vi "pannel-test.vi"() -> ()   [LabVIEW 2019]
uses:
  <vilib>/JDP Science/JSONtext/support/Format JSON Object.vi
  <vilib>/addons/Tools/Unicode/UTF8 Tools.lvlib
  <vilib>/JDP Science/JSONtext/JSONtext.lvlib
panel:
  out "<JSON>":string caption="<JSON>Array"
  out "数组 3":string[][](array[string])
  in  "pannel-list":T1(array[cluster])=[{"node"=[{"ID"="1", "Attribute"="dev", "Action"="", "name"="台灯"}, {"ID"="2", "Attribute"="dev", "Action"="bright-gear", "name"="阅读灯"}], "ID"="0"}, {"node"=[{"ID"="1", "Attribute"="dev", "Action"="", "name"="顶灯"}, {"ID"="2", "Attribute"="dev", "Action"="", "name"="台灯"}], "ID"="1"}, {"node"=[{"ID"="1", "Attribute"="dev", "Action"="open", "name"="窗帘"}, {"ID"="2", "Attribute"="dev", "Action"="close", "name"="窗帘"}], "ID"="2"}]
  out "数组":string[](array[string])
  in  "簇":cluster{"type":string, "payload":string[]}
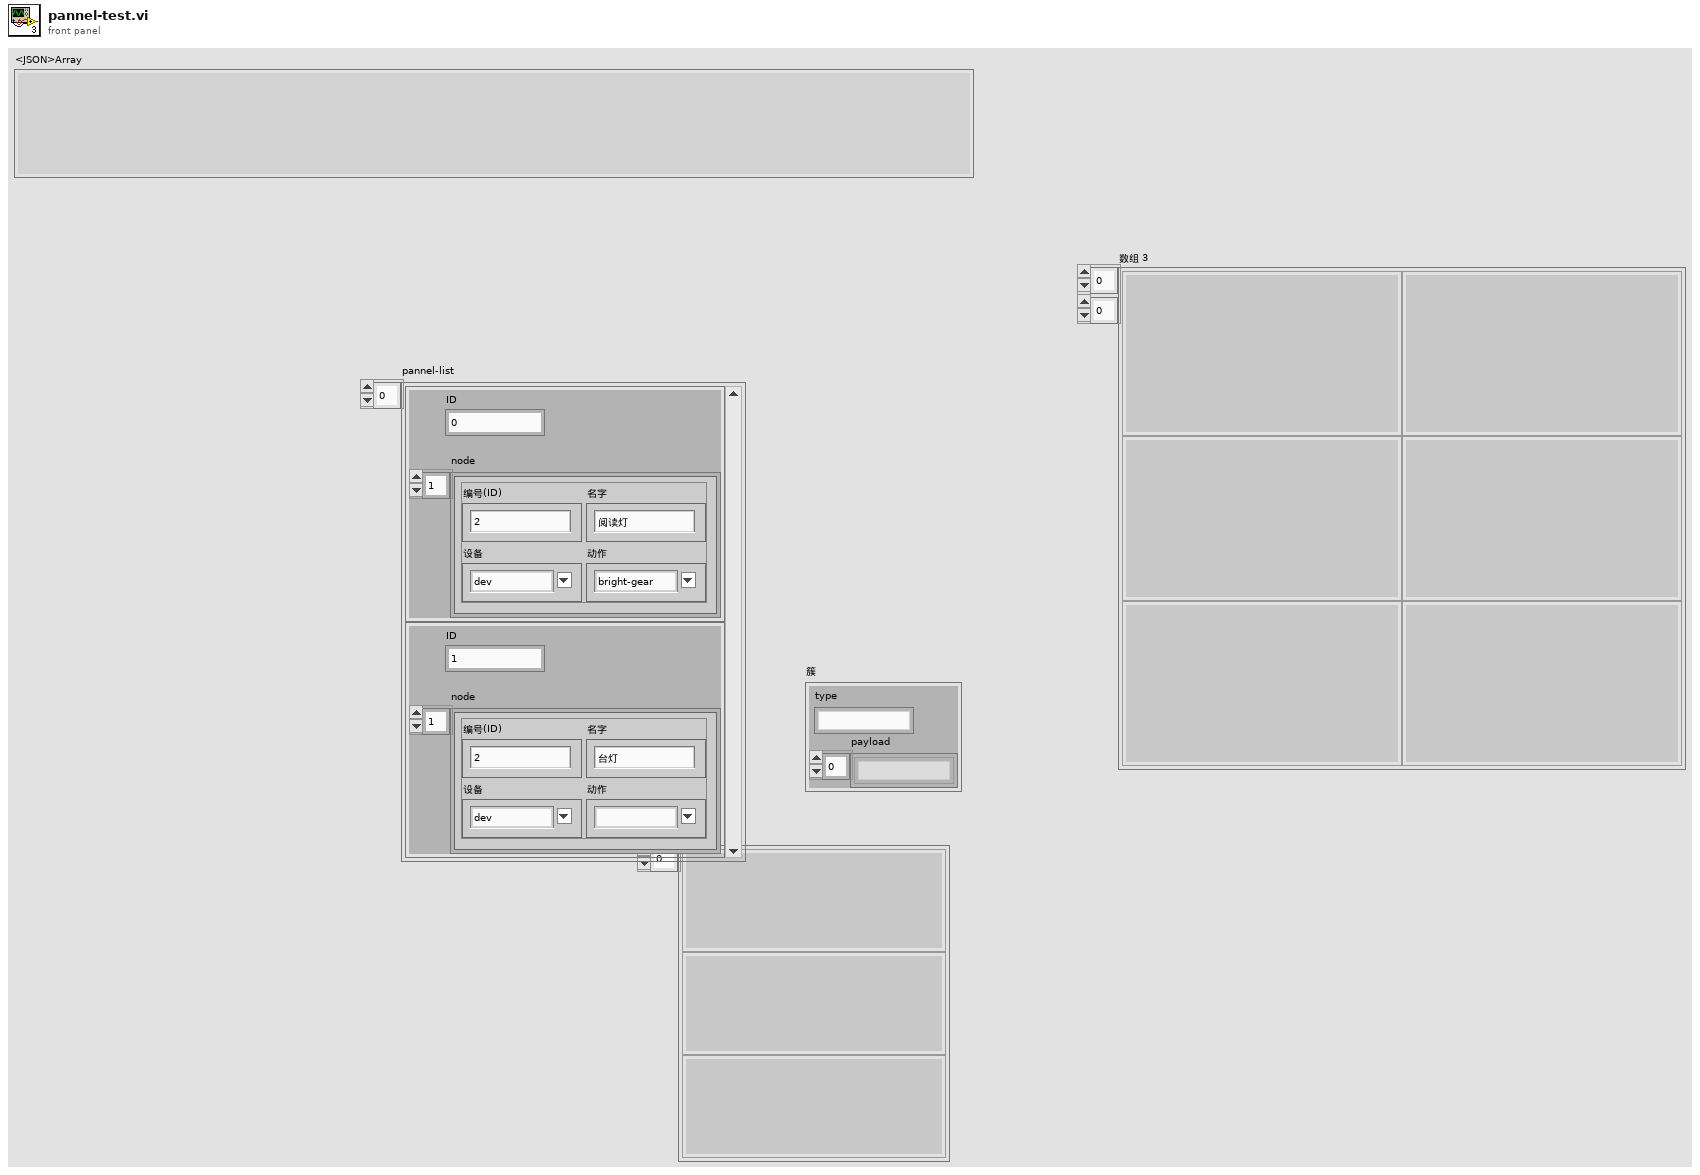
[diagram p1: front panel]
types:
  T1 = cluster{"node":cluster{"ID":string, "Attribute":string, "Action":string, "name":string}[], "ID":string}[]
  T2 = cluster{"ID":string, "Attribute":string, "Action":string, "name":string}[]
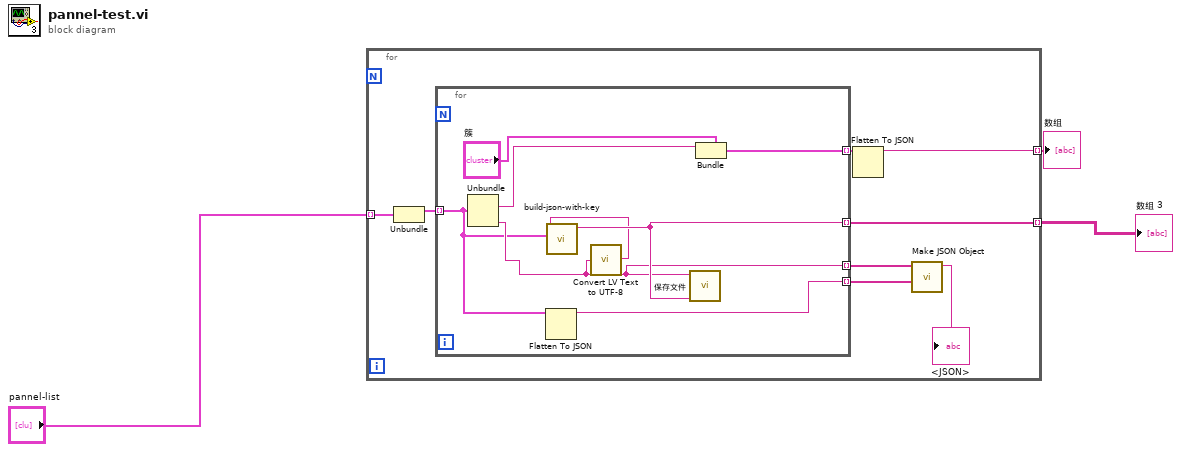
[diagram p0: block diagram]
diagram:
  n1 = for {
    tunnel: "pannel-list" -> [w11] mode=indexing
    tunnel: [w8] -> w3 mode=indexing
    tunnel: [w6] -> w1 mode=indexing
    n2 = Unbundle(w11) -> ("node"=w10:T2)  [unwired: 1 out]
    n3 = for {
      tunnel: w10 -> [w13] mode=indexing
      tunnel: [w18] -> w9 mode=indexing
      tunnel: [w16] -> w6 mode=indexing
      tunnel: [w14] -> w7 mode=indexing
      tunnel: [w12] -> w4 mode=indexing
      n4 = Unbundle(w13) -> ("Attribute"=w17:string, "name"=w14:string)  [unwired: 2 out]
      n5 = Flatten To JSON(anything=w13) -> (JSON string=w12:string)  [unwired: 2 in, 1 out]
      n6 = call <vilib>:"Convert LV Text to UTF-8.vi"("LV Text"=w14) -> ("UTF-8 Text"=w15:string)  [unwired: 13 in, 1 out]
      n7 = call "build-json-with-key.vi"("value"=w13, "key"=w15) -> ("<JSON>First JSON Value\n\n<JSON>"=w16:string)  [unwired: 9 in]
      n8 = call "保存文件.vi"("input"=w16, "文件名"=w14) -> ()  [unwired: 9 in, 1 out]
      n9 = Bundle(cluster="簇", "type"=w17) -> (w18:cluster{"type":string, "payload":string[]})  [unwired: 1 in]
    }
    n10 = Flatten To JSON(anything=w9) -> (JSON string=w8:string)  [unwired: 2 in, 1 out]
    n11 = call <vilib>:"Make JSON Object.vi"("JSON Items"=w4, "Item Names"=w7) -> ("<JSON>"=→"<JSON>":string)  [unwired: 8 in, 1 out]
  }
  "数组" <- w3
  "数组 3" <- w1
